vi "filter mappings by owner.vi"(10 "owner":string, 11 "engine configuration in":refnum<class "base TBM sequencer configuration.lvclass">) -> (2 "module mapping":T1, 3 "engine configuration out":refnum<class "base TBM sequencer configuration.lvclass">)   [LabVIEW 2014, in "base TBM sequencer configuration.lvclass"]
uses:
  base TBM sequencer configuration.lvclass
  Module Mappings.ctl
  <vilib>/NI/Tag Bus/table/mapping specification.ctl
  <vilib>/NI/Tag Bus/tag/Data Type.ctl
  <vilib>/NI/Tag Bus/table/mapping.ctl
  base TBM sequencer configuration.lvclass/base TBM sequencer configuration.ctl
  <vilib>/NI/Tag Bus/tag/tag descriptor.lvclass
  <vilib>/NI/Tag Bus/table/data table.lvlib
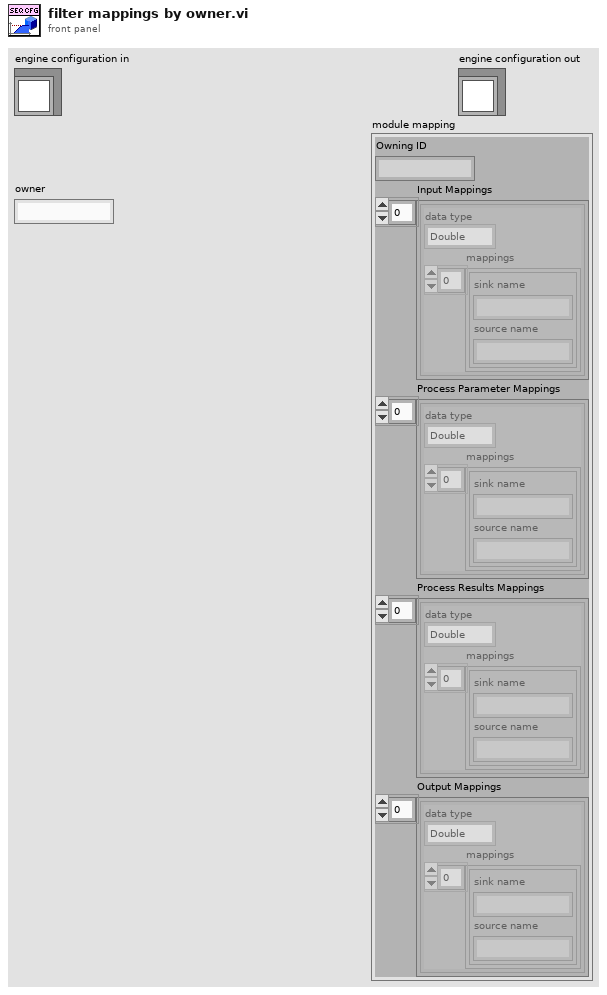
[diagram p1: front panel]
types:
  T1 = typedef "base TBM sequencer configuration.lvclass/Module Mappings.ctl" = cluster{"Owning ID":string, "Input Mappings":T2[], "Process Parameter Mappings":T2[], "Process Results Mappings":T2[], "Output Mappings":T2[]}
  T2 = typedef "tag bus.lvlib/data table.lvlib/mapping specification.ctl" = cluster{"data type":T3, "mappings":T4[]}
  T3 = typedef "tag bus.lvlib/tag descriptor.lvclass/Data Type.ctl" = enum16{"Double", "Single", "I64", "I32", "I16", "I8", "U64", "U32", "U16", "U8", "Boolean", "String", "Array of Double", "Array of Single", "Array of I64", "Array of I32", "Array of I16", "Array of I8", "Array of U64", "Array of U32", "Array of U16", "Array of U8", "Array of Boolean", "Array of String"}
  T4 = typedef "tag bus.lvlib/data table.lvlib/mapping.ctl" = cluster{"sink name":string, "source name":string}
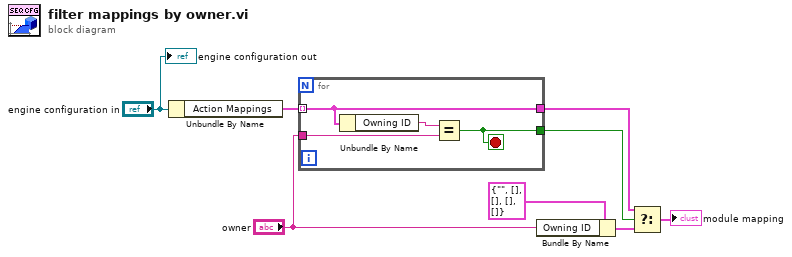
[diagram p0: block diagram]
diagram:
  n1 = Unbundle By Name("engine configuration in") -> ("Action Mappings"=w7:T1[])
  n2 = for {
    tunnel: w7 -> [w10] mode=indexing
    tunnel: "owner" -> [w11]
    tunnel: [w10] -> w6
    tunnel: [w9] -> w1
    stop <- w9 stop-if-true
    n3 = Unbundle By Name(w10) -> ("Owning ID"=w12:string)
    n4 = Equal?(x=w12, y=w11) -> (x = y?=w9:bool)
  }
  n5 = Bundle By Name(cluster=T1 {"Owning ID"="", "Input Mappings"=[], "Process Parameter Mappings"=[], "Process Results Mappings"=[], "Output Mappings"=[]} ("f"), "Owning ID"="owner") -> (w3:T1)
  n6 = Select(t=w6, s=w1, f=w3) -> (s? t:f=→"module mapping":T1)
  "engine configuration out" <- "engine configuration in"
